vi "Read Stream Fields Values.vi"(8 "error in (no error)":errorcluster, 11 "LokiJsonFormatter in":refnum<class "LokiJsonFormatter.lvclass">) -> (0 "error out":errorcluster, 2 "Stream Fields Values":string[](array[string]), 3 "LokiJsonFormatter out":refnum<class "LokiJsonFormatter.lvclass">)   [LabVIEW 2019, in "hse-logger.lvlib" / "LokiJsonFormatter.lvclass"]
uses:
  LokiJsonFormatter.lvclass
  LokiJsonFormatter.lvclass/LokiJsonFormatter.ctl
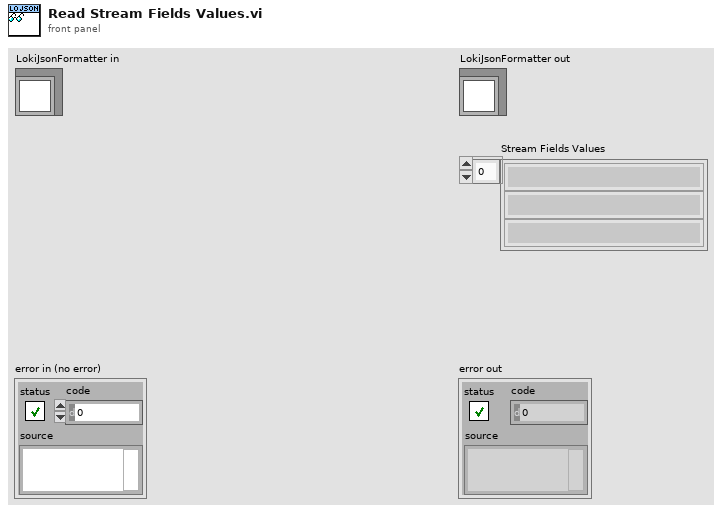
[diagram p1: front panel]
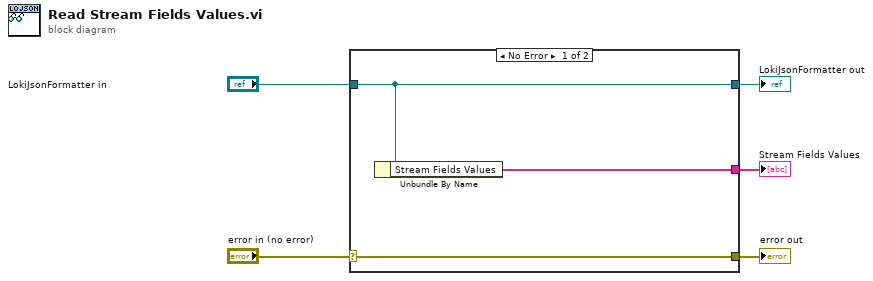
[diagram p0: block diagram]
diagram:
  n1 = case shown="No Error" "error in (no error)" {
    selector: "error in (no error)" -> [w8 w9]
    tunnel: [w8 w9] -> w4
    tunnel: [w7 w10] -> w2
    tunnel: "LokiJsonFormatter in" -> [w7 w10]
    tunnel: [w6 _] -> w1
    frame No Error {
      n2 = Unbundle By Name(w7) -> ("Stream Fields Values"=w6:string[])
    }
    frame Error {
    }
  }
  "error out" <- w4
  "LokiJsonFormatter out" <- w2
  "Stream Fields Values" <- w1
